vi "TempInterpolation.vi"() -> ()   [LabVIEW 2020]
panel:
  in  "Point_grid":dbl[](array[numeric])
  out "element":dbl
  out "Intensity Graph":dbl[][](graph)
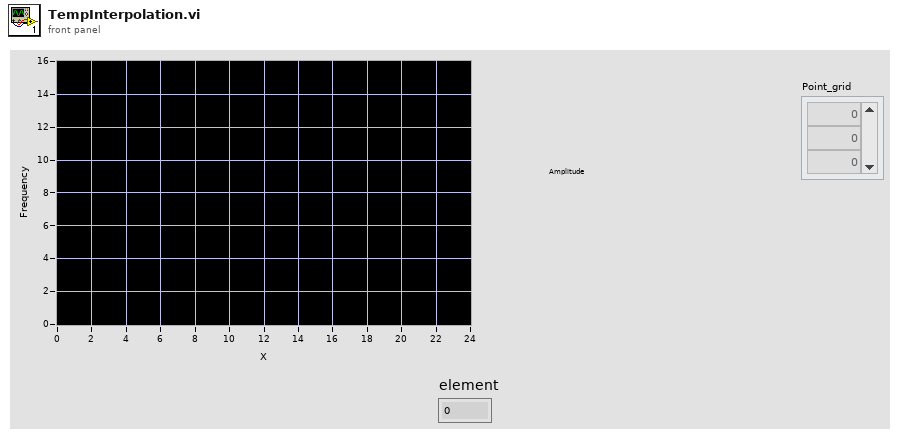
[diagram p1: front panel]
types:
  T1 = typedef "LVPointDoubleTypeDef.ctl" = cluster{"Cursor X":dbl, "Cursor Y":dbl}
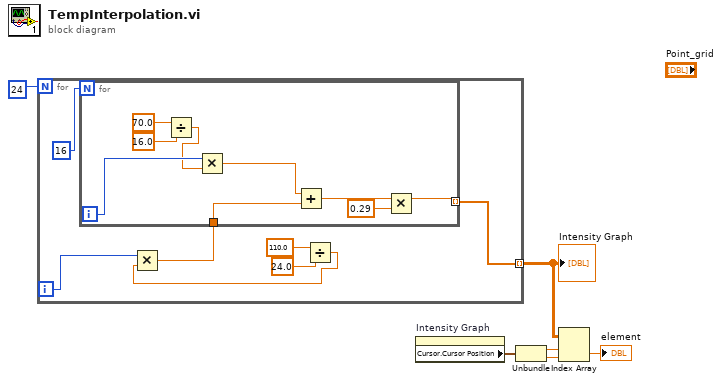
[diagram p0: block diagram]
diagram:
  n1 = for {
    N: 24 -> [_]
    tunnel: [w12] -> w1 mode=indexing
    i -> [w11]
    n2 = Divide(x=110.0, y=24.0) -> (x/y=w7:dbl)
    n3 = Multiply(x=w11, y=w7) -> (x*y=w10:dbl)
    n4 = for {
      N: 16 -> [_]
      tunnel: [w15] -> w12 mode=indexing
      tunnel: w10 -> [w18]
      i -> [w22]
      n5 = Divide(x=70.0, y=16.0) -> (x/y=w19:dbl)
      n6 = Multiply(x=w22, y=w19) -> (x*y=w17:dbl)
      n7 = Add(x=w17, y=w18) -> (x+y=w16:dbl)
      n8 = Multiply(x=w16, y=0.29) -> (x*y=w15:dbl)
    }
  }
  "Intensity Graph" <- w1
  n9 = property on="Intensity Graph" class="IntGraph (strict)"() -> ("Cursor.Cursor Position"=w6:T1)  [unwired: 2 in, 2 out]
  n10 = Unbundle(w6) -> ("Cursor X"=w5:dbl, "Cursor Y"=w4:dbl)
  n11 = Index Array(array=w1, index (row)=w5, index (col)=w4) -> (element=→"element":dbl)
